vi "Perform Lookup Table.vi"(0 "RFmx Instrument Handle In":refnum<k21> caption="Instrument Handle In", 1 "Selector String":string, 5 "SG Instrument Handle In":refnum<k15>, 7 "Reference Waveform":T2={"Name"="Wfm", "Data"=refnum, "Signal Bandwidth (Hz)"=0.0, "PAPR (dB)"=0.0, "Burst Length (s)"=0.0, "Sample Rate"=0.0, "Burst Start Locations"=[], "Burst Stop Locations"=[], "Idle Duration Present?"=FALSE, "Runtime Scaling"=0.0, "Script"=""} {"Runtime Scaling" format="%#_6p"; "Sample Rate" format="%#_6p"; "Burst Length (s)" format="%#_6p"; "PAPR (dB)" format="%.2f"; "Signal Bandwidth (Hz)" format="%#_6p"}, 11 "error in (no error)":errorcluster) -> (4 "RFmx Instrument Handle Out":refnum<k21> caption="Instrument Handle Out", 6 "SG Instrument Handle Out":refnum<k15>, 8 "Lookup Table Results":T1={"Predistorted Waveform"={"Name"="Wfm", "Data"=refnum, "Signal Bandwidth (Hz)"=0.0, "PAPR (dB)"=0.0, "Burst Length (s)"=0.0, "Sample Rate"=0.0, "Burst Start Locations"=[], "Burst Stop Locations"=[], "Idle Duration Present?"=FALSE, "Runtime Scaling"=0.0, "Script"=""}, "Input Powers (dBm)"=[], "Complex Gains (dB)"=[], "Power Results"={"Waveform Power Offset (dB)"=-1.0, "Waveform True PAPR (dB)"=0.0, "Training Power (dBm)"=0.0}} {"Power Results"."Training Power (dBm)" format="%.2f"; "Power Results"."Waveform True PAPR (dB)" format="%.2f"; "Power Results"."Waveform Power Offset (dB)" format="%.2f"; "Predistorted Waveform"."Runtime Scaling" format="%#_6p"; "Predistorted Waveform"."Sample Rate" format="%#_6p"; "Predistorted Waveform"."Burst Length (s)" format="%#_6p"; "Predistorted Waveform"."PAPR (dB)" format="%.2f"; "Predistorted Waveform"."Signal Bandwidth (Hz)" format="%#_6p"}, 15 "error out":errorcluster)   [LabVIEW 2019, in "RFmxDPD.lvlib"]
doc: "Acquires the incoming signal, trains the DPD model, applies the lookup table to the reference waveform, and downloads the predistorted waveform to the generator. If generation is in progress when this function is called, generation will resume with the predistorted waveform."
uses:
  RFmxDPD.lvlib
  Common/Waveform.ctl
  Typedefs/Lookup Table Results.ctl
  <vilib>/RFmx/SpecAn/mx/RFmxSpecAn.llb/RFmxSpecAn DPD Fetch Lookup Table.vi
  SG/SG.lvlib
  Common/Common.lvlib
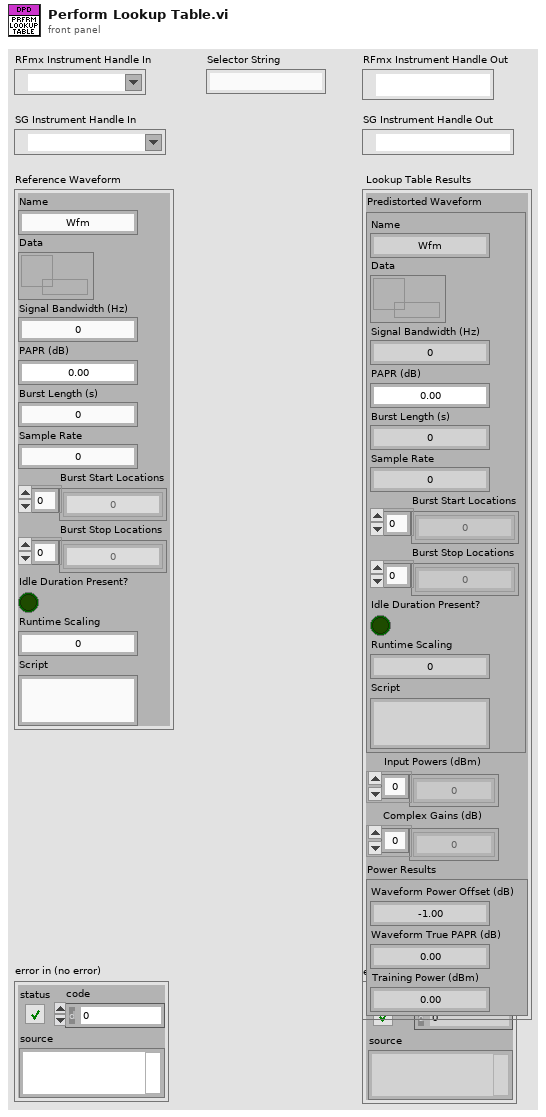
[diagram p1: front panel]
types:
  T1 = typedef "RFmxDPD.lvlib/Lookup Table Results.ctl" = cluster{"Predistorted Waveform":T2, "Input Powers (dBm)":sgl[], "Complex Gains (dB)":csg[], "Power Results":cluster{"Waveform Power Offset (dB)":dbl, "Waveform True PAPR (dB)":dbl, "Training Power (dBm)":dbl}}
  T2 = typedef "Common.lvlib/Waveform.ctl" = cluster{"Name":string, "Data":refnum<data-value>, "Signal Bandwidth (Hz)":dbl, "PAPR (dB)":dbl, "Burst Length (s)":dbl, "Sample Rate":dbl, "Burst Start Locations":i32[], "Burst Stop Locations":i32[], "Idle Duration Present?":bool, "Runtime Scaling":dbl, "Script":string}
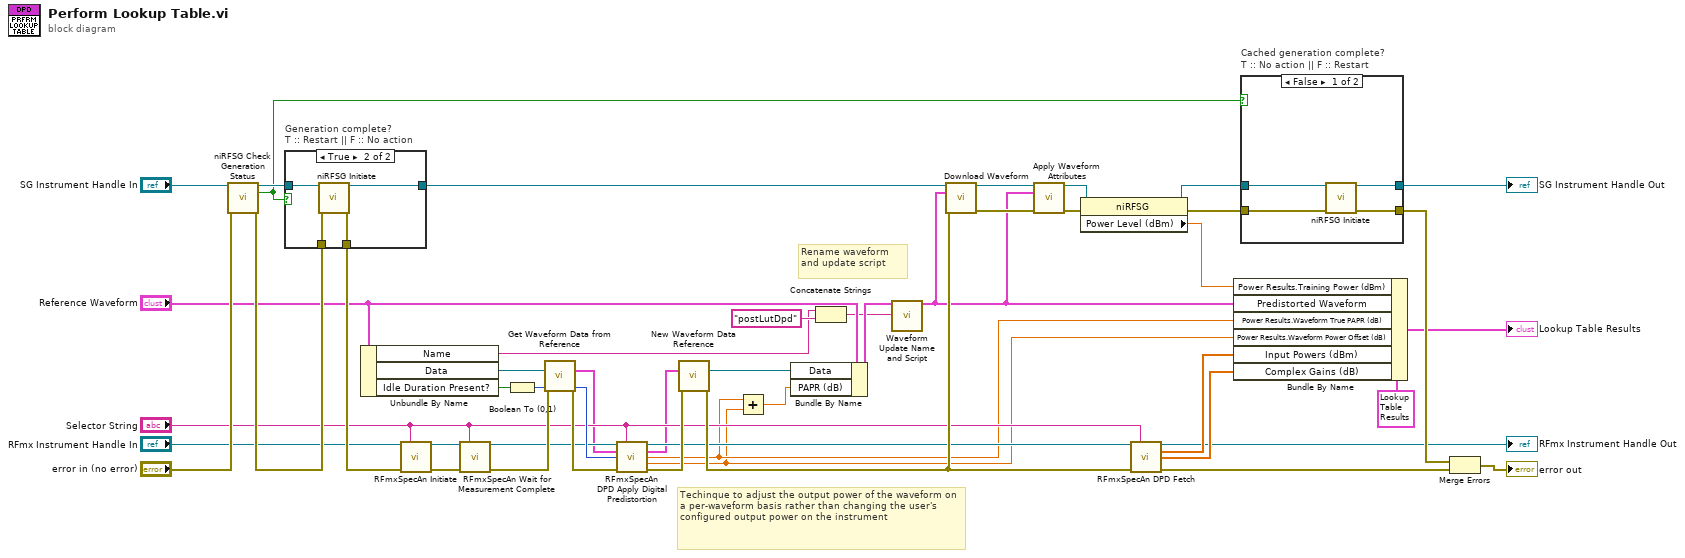
[diagram p0: block diagram]
diagram:
  # "Techinque to adjust the output power of the waveform on a per-waveform basis rather than changing the user's configured output power on the instrument"
  # "Rename waveform and update script"
  n1 = call <instrlib>:"niRFSG Check Generation Status.vi"("instrument handle"="SG Instrument Handle In", "error in"="error in (no error)") -> ("instrument handle out"=w23:refnum<k15>, "done?"=w20:bool, "error out"=w48:errorcluster)  [unwired: 11 in]
  n2 = case "Generation complete?\nT :: Restart || F :: No action" shown="True" w20 {
    tunnel: w48 -> [w50 w54]
    tunnel: w23 -> [w49 w52]
    tunnel: [w49 w51] -> w22
    tunnel: [w50 w53] -> w35
    frame False {
    }
    frame True {
      n3 = call <instrlib>:"niRFSG Initiate.vi"("instrument handle"=w52, "error in"=w54) -> ("instrument handle out"=w51:refnum<k15>, "error out"=w53:errorcluster)  [unwired: 12 in]
    }
  }
  n4 = Unbundle By Name("Reference Waveform") -> ("Name"=w17:string, "Data"=w33:refnum<data-value>, "Idle Duration Present?"=w3:bool)
  n5 = call <vilib>:"RFmxSpecAn Initiate.vi"("Instrument Handle In"="RFmx Instrument Handle In", "Selector String"="Selector String", "error in (no error)"=w35) -> ("Instrument Handle Out"=w16:refnum<k21>, "error out"=w47:errorcluster)  [unwired: 10 in, 1 out]
  n6 = call <vilib>:"RFmxSpecAn Wait for Measurement Complete.vi"("Instrument Handle In"=w16, "Selector String"="Selector String", "error in (no error)"=w47) -> ("Instrument Handle Out"=w15:refnum<k21>, "error out"=w39:errorcluster)  [unwired: 11 in]
  n7 = Boolean To (0,1)(Boolean=w3) -> (0, 1=w32:i16)
  n8 = call "Get Waveform Data from Reference.vi"("Waveform Data Reference"=w33, "error in (no error)"=w39) -> ("Waveform Data"=w5:cluster{"t0":dbl, "dt":dbl, "y":csg[]}, "error out"=w40:errorcluster)  [unwired: 12 in]
  n9 = call <vilib>:"RFmxSpecAn DPD Apply Digital Predistortion.vi"("Instrument Handle In"=w15, "Selector String"="Selector String", "Waveform In"=w5, "Idle Duration Present"=w32, "error in (no error)"=w40) -> ("Instrument Handle Out"=w18:refnum<k21>, "Waveform Out"=w4:cluster{"x0":dbl, "dx":dbl, "y":csg[]}, "PAPR (dB)"=w8:dbl, "Power Offset (dB)"=w7:dbl, "error out"=w38:errorcluster)  [unwired: 6 in]
  n10 = call "New Waveform Data Reference.vi"("Waveform Data"=w4, "error in (no error)"=w38) -> ("Waveform Data Reference"=w6:refnum<data-value>, "error out"=w37:errorcluster)  [unwired: 12 in]
  n11 = Add(x=w8, y=w7) -> (x+y=w9:dbl)
  n12 = Bundle By Name(cluster="Reference Waveform", "Data"=w6, "PAPR (dB)"=w9) -> (w21:T2)
  n13 = Concatenate Strings(w17, "postLutDpd" ("string")) -> (w1:string)
  n14 = call "Waveform Update Name and Script.vi"("Waveform in"=w21, "New Waveform Name"=w1) -> ("Waveform out"=w2:T2)  [unwired: 13 in]
  n15 = call "Download Waveform.vi"("RFSG handle"=w22, "Waveform In"=w2, "error in (no error)"=w37) -> ("RFSG handle out"=w13:refnum<k15>, "error out"=w43:errorcluster)  [unwired: 11 in]
  n16 = call "Apply Waveform Attributes.vi"("RFSG Session In"=w13, "Waveform"=w2, "error in (no error)"=w43) -> ("RFSG Session Out"=w12:refnum<k15>, "error out"=w42:errorcluster)  [unwired: 11 in]
  n17 = property class="niRFSG"(reference=w12, error in=w42) -> (reference out=w11:refnum<k15>, error out=w41:errorcluster, "Power Level (dBm)"=w10:dbl)
  n18 = call-poly <vilib>:"RFmxSpecAn DPD Fetch.vi"("Instrument Handle In"=w18, "Selector String"="Selector String", "error in (no error)"=w37) -> ("Instrument Handle Out"=→"RFmx Instrument Handle Out":refnum<k21>, "Input Powers"=w29:sgl[], "Complex Gains"=w28:csg[], "error out"=w45:errorcluster)  [unwired: 9 in]
  n19 = Bundle By Name(cluster=T1 {"Predistorted Waveform"={"Name"="Wfm", "Data"=refnum, "Signal Bandwidth (Hz)"=0.0, "PAPR (dB)"=0.0, "Burst Length (s)"=0.0, "Sample Rate"=0.0, "Burst Start Locations"=[], "Burst Stop Locations"=[], "Idle Duration Present?"=FALSE, "Runtime Scaling"=0.0, "Script"=""}, "Input Powers (dBm)"=[], "Complex Gains (dB)"=[], "Power Results"={"Waveform Power Offset (dB)"=-1.0, "Waveform True PAPR (dB)"=0.0, "Training Power (dBm)"=0.0}} ("Lookup Table Results"), "Power Results.Training Power (dBm)"=w10, "Predistorted Waveform"=w2, "Power Results.Waveform True PAPR (dB)"=w8, "Power Results.Waveform Power Offset (dB)"=w7, "Input Powers (dBm)"=w29, "Complex Gains (dB)"=w28) -> (→"Lookup Table Results":T1)
  n20 = case "Cached generation complete?\nT :: No action || F :: Restart" shown="False" w20 {
    tunnel: [w56 w59] -> w31
    tunnel: [w58 w60] -> w46
    tunnel: w11 -> [w55 w59]
    tunnel: w41 -> [w57 w60]
    frame False {
      n21 = call <instrlib>:"niRFSG Initiate.vi"("instrument handle"=w55, "error in"=w57) -> ("instrument handle out"=w56:refnum<k15>, "error out"=w58:errorcluster)  [unwired: 12 in]
    }
    frame True {
    }
  }
  "SG Instrument Handle Out" <- w31
  n22 = Merge Errors(w46, w45) -> (→"error out":errorcluster)
